vi "GetCarImage.vi"(8 "Error In":errorcluster, 11 "reference in":refnum<class "Hatchback.lvclass">) -> (0 "Error Out":errorcluster, 2 "Image Path":path, 3 "reference out":refnum<class "Hatchback.lvclass">)   [LabVIEW 2024, in "Hatchback.lvclass"]
uses:
  Hatchback.lvclass
  Hatchback.lvclass/Hatchback.ctl
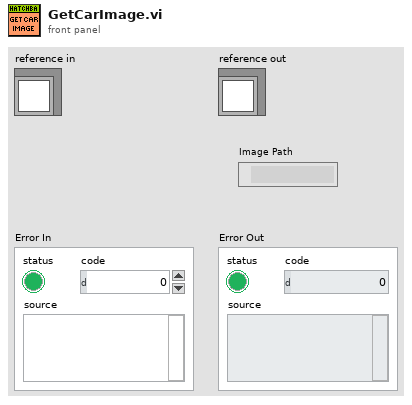
[diagram p1: front panel]
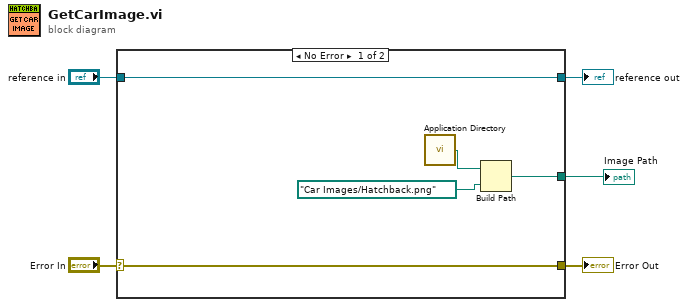
[diagram p0: block diagram]
diagram:
  n1 = case shown="No Error" "Error In" {
    selector: "Error In" -> [w9 w12]
    tunnel: [w9 w12] -> w4
    tunnel: [w10 w11] -> w2
    tunnel: "reference in" -> [w10 w11]
    tunnel: [w6 _] -> w1
    frame No Error {
      n2 = call <vilib>:"Application Directory.vi"() -> ("Application Directory"=w8:path)
      n3 = Build Path(base path=w8, name or relative path=path "Car Images/Hatchback.png") -> (appended path=w6:path)
    }
    frame Error {
    }
  }
  "Error Out" <- w4
  "reference out" <- w2
  "Image Path" <- w1
